vi "FPGA1_EPTDigChannels_eDIDS.vi"(0 "9411 Inputs":cluster{"9411-1/DI5:0":u8, "9411-2/DI5:0":u8}, 1 "9411 Invert Commands":T2, 2 "9411-1.FilterValues":T1, 3 "9411-2.FilterValues":T1) -> (6 "9411-1.0.PPWData":T3, 7 "9411-1.4.PPWData":T3, 8 "9411-1.1.PPWData":T3, 9 "9411-1.5.PPWData":T3, 10 "9411-1.2.PPWData":T3, 11 "9411-2.0.PPWData":T3, 12 "9411-1.3.PPWData":T3, 13 "9411-2.1.PPWData":T3, 14 "9411-2.2.PPWData":T3, 15 "9411-2.3.PPWData":T3, 16 "9411-2.4.PPWData":T3, 17 "9411-2.5.PPWData":T3, 18 "9411-1.DigitalTriggers":bool[](array[boolean]), 19 "9411-2.DigitalTriggers":bool[](array[boolean]))   [LabVIEW 2015, in "ECS-FPGA.lvlib"]
uses:
  ECS-FPGA.lvlib
  <vilib>/Powertrain Controls/Device Drivers/Tools/FPGA/ppw_reva.vi
  <vilib>/Powertrain Controls/Device Drivers/Tools/FPGA/filt_int_reva.vi
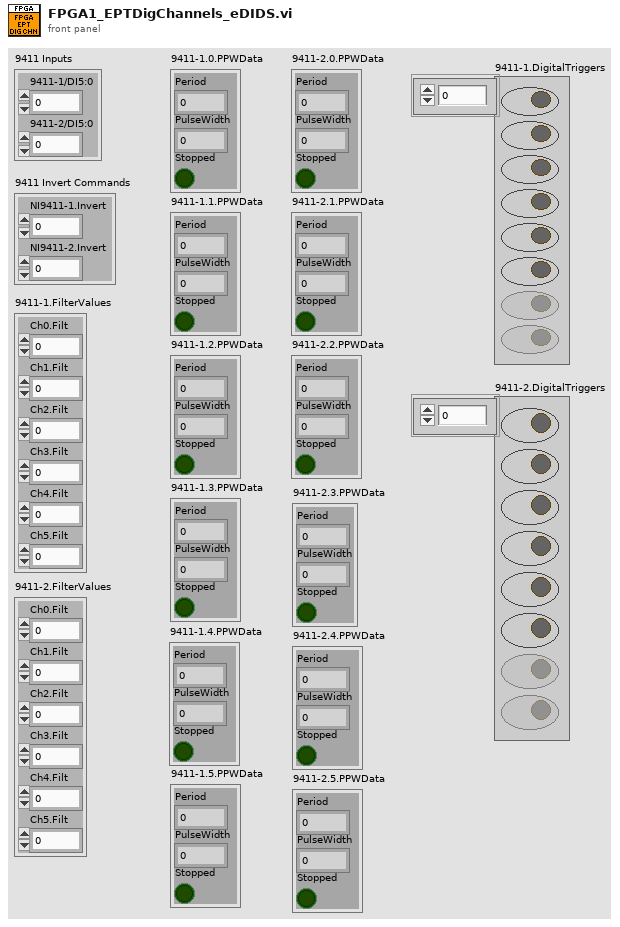
[diagram p1: front panel]
types:
  T1 = cluster{"Ch0.Filt":u16, "Ch1.Filt":u16, "Ch2.Filt":u16, "Ch3.Filt":u16, "Ch4.Filt":u16, "Ch5.Filt":u16}
  T2 = cluster{"NI9411-1.Invert":u8, "NI9411-2.Invert":u8}
  T3 = cluster{"Period":u32, "PulseWidth":u32, "Stopped":bool}
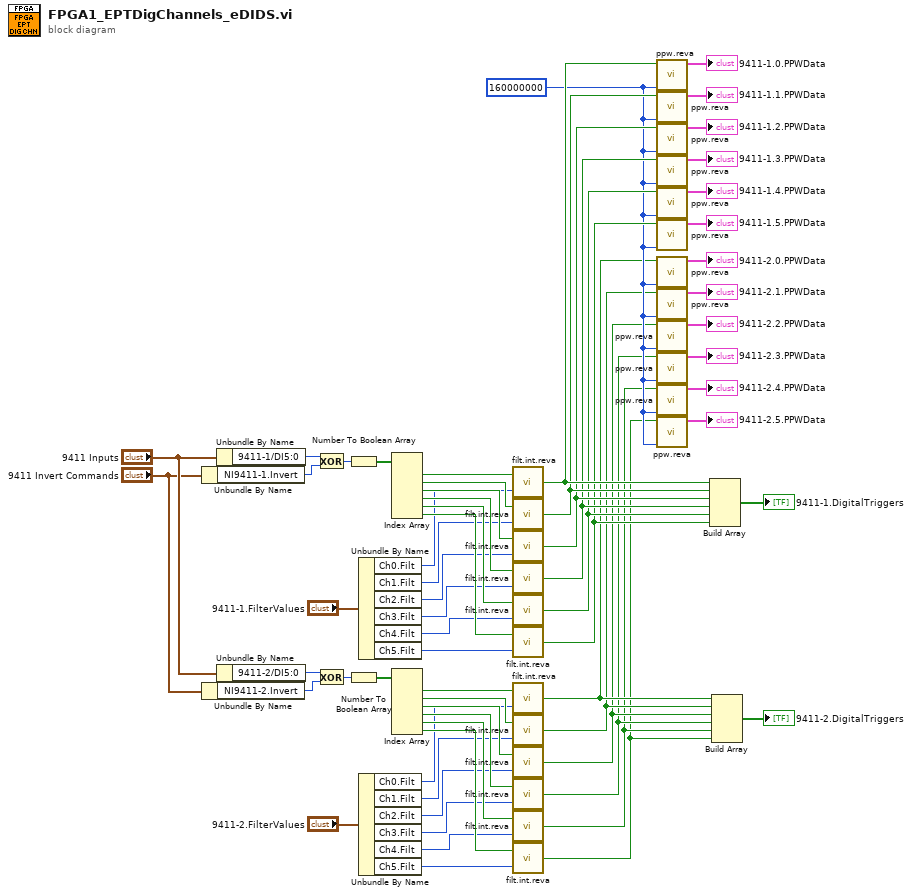
[diagram p0: block diagram]
diagram:
  w28 = u32 160000000 ("StopValue")
  n1 = Unbundle By Name("9411 Invert Commands") -> ("NI9411-1.Invert"=w13:u8)
  n2 = Unbundle By Name("9411 Invert Commands") -> ("NI9411-2.Invert"=w9:u8)
  n3 = Unbundle By Name("9411 Inputs") -> ("9411-1/DI5:0"=w14:u8)
  n4 = Unbundle By Name("9411 Inputs") -> ("9411-2/DI5:0"=w12:u8)
  n5 = Exclusive Or(1:w13, 2:w14) -> (0:w48:u8)
  n6 = Exclusive Or(1:w9, 2:w12) -> (0:w42:u8)
  n7 = Number To Boolean Array(number=w48) -> (Boolean array=w49:bool[])
  n8 = Number To Boolean Array(number=w42) -> (Boolean array=w41:bool[])
  n9 = Unbundle By Name("9411-1.FilterValues") -> ("Ch0.Filt"=w26:u16, "Ch1.Filt"=w25:u16, "Ch2.Filt"=w24:u16, "Ch3.Filt"=w23:u16, "Ch4.Filt"=w22:u16, "Ch5.Filt"=w21:u16)
  n10 = Unbundle By Name("9411-2.FilterValues") -> ("Ch0.Filt"=w20:u16, "Ch1.Filt"=w19:u16, "Ch2.Filt"=w18:u16, "Ch3.Filt"=w17:u16, "Ch4.Filt"=w16:u16, "Ch5.Filt"=w15:u16)
  n11 = Index Array(array=w49) -> (element #1=w50:bool, element #2=w51:bool, element #3=w52:bool, element #4=w53:bool, element #5=w54:bool, element #6=w55:bool)  [unwired: 6 in]
  n12 = Index Array(array=w41) -> (element #1=w40:bool, element #2=w39:bool, element #3=w38:bool, element #4=w37:bool, element #5=w36:bool, element #6=w35:bool)  [unwired: 6 in]
  n13 = call "filt.int.reva.vi"("FiltValue"=w26, "InpSig"=w50) -> ("OutSig"=w63:bool)
  n14 = call "filt.int.reva.vi"("FiltValue"=w25, "InpSig"=w51) -> ("OutSig"=w47:bool)
  n15 = call "filt.int.reva.vi"("FiltValue"=w24, "InpSig"=w52) -> ("OutSig"=w46:bool)
  n16 = call "filt.int.reva.vi"("FiltValue"=w23, "InpSig"=w53) -> ("OutSig"=w45:bool)
  n17 = call "filt.int.reva.vi"("FiltValue"=w22, "InpSig"=w54) -> ("OutSig"=w44:bool)
  n18 = call "filt.int.reva.vi"("FiltValue"=w21, "InpSig"=w55) -> ("OutSig"=w43:bool)
  n19 = call "filt.int.reva.vi"("FiltValue"=w20, "InpSig"=w40) -> ("OutSig"=w6:bool)
  n20 = call "filt.int.reva.vi"("FiltValue"=w19, "InpSig"=w39) -> ("OutSig"=w5:bool)
  n21 = call "filt.int.reva.vi"("FiltValue"=w18, "InpSig"=w38) -> ("OutSig"=w4:bool)
  n22 = call "filt.int.reva.vi"("FiltValue"=w17, "InpSig"=w37) -> ("OutSig"=w3:bool)
  n23 = call "filt.int.reva.vi"("FiltValue"=w16, "InpSig"=w36) -> ("OutSig"=w2:bool)
  n24 = call "filt.int.reva.vi"("FiltValue"=w15, "InpSig"=w35) -> ("OutSig"=w1:bool)
  n25 = call "ppw.reva.vi"("StopValue"=w28, "InpSig"=w63) -> ("PPWData"=→"9411-1.0.PPWData":T3)  [unwired: 2 in, 3 out]
  n26 = call "ppw.reva.vi"("StopValue"=w28, "InpSig"=w47) -> ("PPWData"=→"9411-1.1.PPWData":T3)  [unwired: 2 in, 3 out]
  n27 = call "ppw.reva.vi"("StopValue"=w28, "InpSig"=w46) -> ("PPWData"=→"9411-1.2.PPWData":T3)  [unwired: 2 in, 3 out]
  n28 = call "ppw.reva.vi"("StopValue"=w28, "InpSig"=w45) -> ("PPWData"=→"9411-1.3.PPWData":T3)  [unwired: 2 in, 3 out]
  n29 = call "ppw.reva.vi"("StopValue"=w28, "InpSig"=w44) -> ("PPWData"=→"9411-1.4.PPWData":T3)  [unwired: 2 in, 3 out]
  n30 = call "ppw.reva.vi"("StopValue"=w28, "InpSig"=w43) -> ("PPWData"=→"9411-1.5.PPWData":T3)  [unwired: 2 in, 3 out]
  n31 = call "ppw.reva.vi"("StopValue"=w28, "InpSig"=w6) -> ("PPWData"=→"9411-2.0.PPWData":T3)  [unwired: 2 in, 3 out]
  n32 = call "ppw.reva.vi"("StopValue"=w28, "InpSig"=w5) -> ("PPWData"=→"9411-2.1.PPWData":T3)  [unwired: 2 in, 3 out]
  n33 = call "ppw.reva.vi"("StopValue"=w28, "InpSig"=w4) -> ("PPWData"=→"9411-2.2.PPWData":T3)  [unwired: 2 in, 3 out]
  n34 = call "ppw.reva.vi"("StopValue"=w28, "InpSig"=w3) -> ("PPWData"=→"9411-2.3.PPWData":T3)  [unwired: 2 in, 3 out]
  n35 = call "ppw.reva.vi"("StopValue"=w28, "InpSig"=w2) -> ("PPWData"=→"9411-2.4.PPWData":T3)  [unwired: 2 in, 3 out]
  n36 = call "ppw.reva.vi"("StopValue"=w28, "InpSig"=w1) -> ("PPWData"=→"9411-2.5.PPWData":T3)  [unwired: 2 in, 3 out]
  n37 = Build Array(w63, w47, w46, w45, w44, w43) -> (→"9411-1.DigitalTriggers":bool[])
  n38 = Build Array(w6, w5, w4, w3, w2, w1) -> (→"9411-2.DigitalTriggers":bool[])
